vi "WPI_SimpleGyro_Loop.vi"(8 "error in":errorcluster, 11 "SimpleGyroDevRef":T1 {"Sample Rate" min=0.25 max=100.0 step=0.25}) -> (0 "error out":errorcluster)   [LabVIEW 2015, in "FRC Gyro and Accel.lvlib"]
doc: "Periodically reads the SimpleGyro and makes data available to your robot project. Place this block within PeriodicTasks.vi."
uses:
  FRC Gyro and Accel.lvlib
  WPI_SimpleGyroDevRef.ctl
  <vilib>/Rock Robotics/SystemInterfaces/spilib/spi_bus.ctl
  <vilib>/Rock Robotics/WPI/SPI/WPI_SPIDevRef.ctl
  <vilib>/Platform/TimedLoop/XDataNode/timing_clust.ctl
  <vilib>/Platform/TimedLoop/XDataNode/nitl_modes.ctl
  <vilib>/Platform/TimedLoop/XDataNode/wakeup.ctl
  <vilib>/platform/TimedLoop/XDataNode/XDataNode.xnode
  <vilib>/Platform/TimedLoop/XDataNode/XDNodeRunTimeDep.lvlib
  <vilib>/ptbypt/NI_PtbyPt.lvlib
panel:
  out "Rate":dbl
  out "Device Found":bool
  out "Offset":dbl
  out "mean 2":dbl format="%0.2f"
  out "Angle":dbl
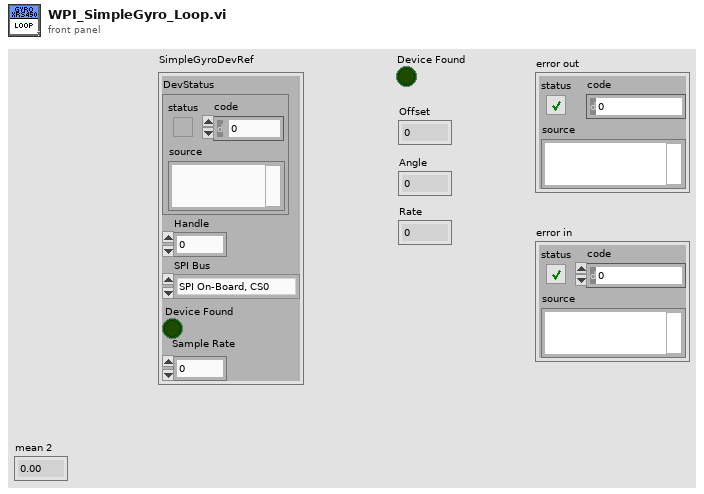
[diagram p1: front panel]
types:
  T1 = typedef "FRC Gyro and Accel.lvlib/WPI_SimpleGyroDevRef.ctl" = cluster{"DevStatus":errorcluster, "Handle":i32, "SPI Bus":T2, "Device Found":bool, "Sample Rate":dbl}
  T2 = typedef "spi_bus.ctl" = enum16{"SPI On-Board, CS0", "SPI On-Board, CS1", "SPI On-Board, CS2", "SPI On-Board, CS3", "SPI MXP", "Invalid"}
  T3 = typedef "WPI_SPIDevRef.ctl" = cluster{"DevStatus":errorcluster, "Handle":i32, "SPI Bus":T2}
  T4 = typedef "XDNodeRunTimeDep.lvlib/timing_clust.ctl" = cluster{"Expected End [f-1]":u64, "Actual End [f-1]":u64, "Finished Late? [f-1]":bool, "Expected End [i-1]":u64, "Actual End [i-1]":u64, "Finished Late? [i-1]":bool, "Expected Start [i]":u64, "Actual Start [i]":u64, "Expected Start [f]":u64, "Actual Start [f]":u64, "Source Name":string, "Structure Name":string, "Period":i64, "Deadline":i64, "Offset":i64, "Start":i64, "Priority":i32, "Timeout":i32, "Mode":T5, "Wakeup Reason":T6, "Error":errorcluster, "Source Type":string, "Secondary Source Type":string, "Global End Time":u64, "Global Start Time":u64, "Frame Duration":u64, "Iteration Duration":u64, "Assigned CPU":i32, "I/O Scan Engine Mode":u32}
  T5 = typedef "XDNodeRunTimeDep.lvlib/nitl_modes.ctl" = enum32{"No Change", "Process missed periods, maintain original phase", "Discard missed periods, maintain original phase", "Process missed periods, ignore original phase", "Discard missed periods, ignore original phase"}
  T6 = typedef "XDNodeRunTimeDep.lvlib/wakeup.ctl" = enum32{"Normal", "Aborted", "Asynchronous wakeup", "Timing source error", "Timed loop error", "Timeout"}
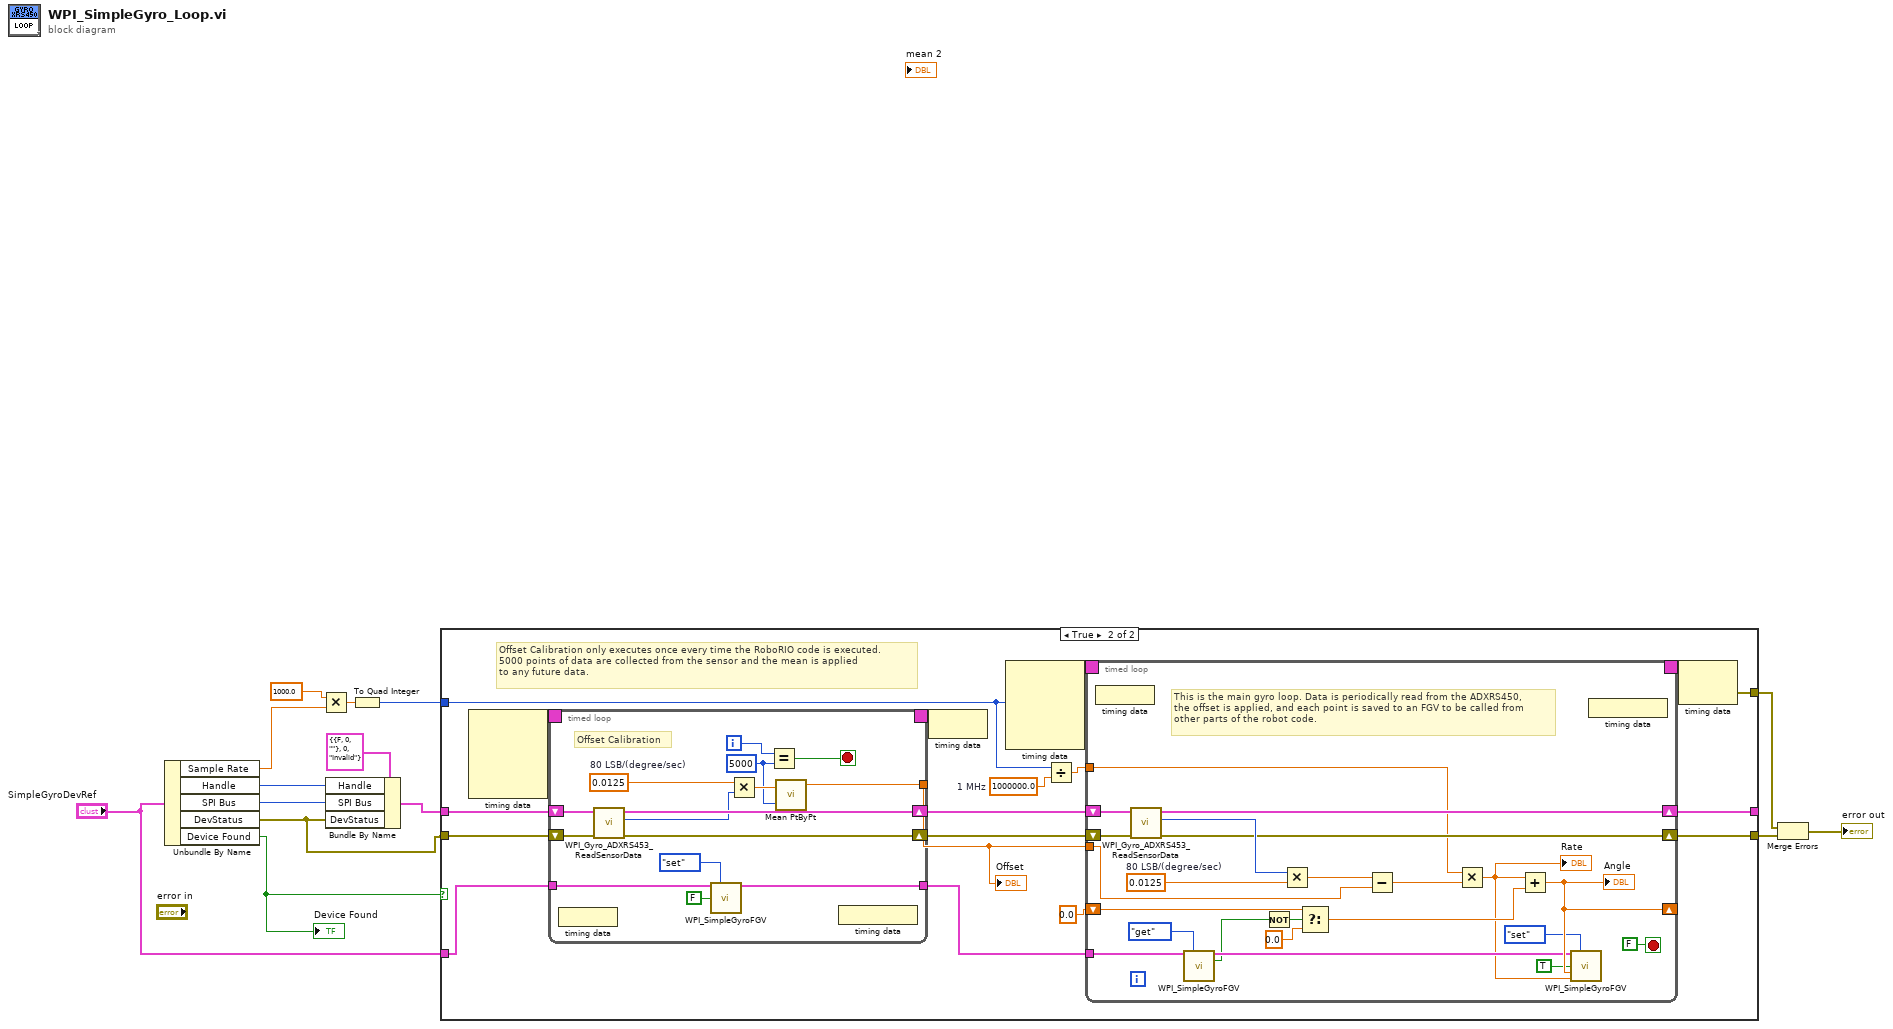
[diagram p0: block diagram]
diagram:
  n1 = Unbundle By Name("SimpleGyroDevRef") -> ("Sample Rate"=w4:dbl, "Handle"=w13:i32, "SPI Bus"=w12:T2, "DevStatus"=w1:errorcluster, "Device Found"=w11:bool)
  "Device Found" <- w11
  n2 = Multiply(x=1000.0 ("y"), y=w4) -> (x*y=w10:dbl)
  n3 = Bundle By Name(cluster=T3 {"DevStatus"={"status"=FALSE, "code"=0, "source"=""}, "Handle"=0, "SPI Bus"=enum."Invalid"} ("SPIDevRef out"), "Handle"=w13, "SPI Bus"=w12, "DevStatus"=w1) -> (w2:T3)
  n4 = To Quad Integer(1:w10) -> (0:w9:i64)
  n5 = case shown="True" w11 {
    tunnel: w2 -> [w16 w23]
    tunnel: w1 -> [w15 w22]
    tunnel: [w15 w32] -> w7
    tunnel: [w16 w31] -> _
    tunnel: w9 -> [_ w29]
    tunnel: "SimpleGyroDevRef" -> [_ w18]
    tunnel: [_ w28] -> w6
    frame False {
    }
    frame True {
      w26 = 1000000.0  # 1 MHz
      # "Offset Calibration only executes once every time the RoboRIO code is executed.\n5000 points of data are collected from the sensor and the mean is applied\nto any future data."
      n6 = node-c288() -> (w25:T4)  [unwired: 4 in]
      n7 = timed-loop {
        shift-right: [w47] -> w21
        shift-left: w23 -> [w49]
        shift-right: [w44] -> w20
        shift-left: w22 -> [w48]
        timing: w25 -> [_]
        timing-out: [_] -> w24
        tunnel: [w42] -> w19
        tunnel: w18 -> [w37]
        tunnel: [w35] -> w17
        i -> [w41]
        stop <- w39 stop-if-true
        w40 = 5000 ("y")
        w45 = 0.0125  # 80 LSB/(degree/sec)
        # "Offset Calibration"
        n8 = node-c288() -> ()  [unwired: 1 in]
        n9 = call "WPI_Gyro_ADXRS453_ReadSensorData.vi"("error in (no error)"=w48, "SPIDevRef in"=w49) -> ("error out"=w44:errorcluster, "Sensor Data (n-1)"=w46:i16, "SPIDevRef out"=w47:T3)  [unwired: 5 in, 2 out]
        n10 = call "WPI_SimpleGyroFGV.vi"("SimpleGyroDevRef"=w37, "Operation"=enum16{"set", "get"}."set", "Calibrated"=FALSE) -> ("SimpleGyroDevRef"=w35:T1)  [unwired: 8 in, 4 out]
        n11 = Multiply(x=w45, y=w46) -> (x*y=w43:dbl)
        n12 = Equal?(x=w41, y=w40) -> (x = y?=w39:bool)
        n13 = call <vilib>:"Mean PtByPt.vi"("x"=w43, "sample length"=w40) -> ("mean"=w42:dbl)  [unwired: 2 in, 1 out]
        n14 = node-c288() -> ()  [unwired: 1 out]
      }
      "Offset" <- w19
      n15 = node-c288(w24) -> ()
      n16 = node-c288(w29) -> (w34:T4)  [unwired: 3 in]
      n17 = Divide(x=w29, y=w26) -> (x/y=w30:dbl)
      n18 = timed-loop {
        shift-right: [w74] -> w31
        shift-left: w21 -> [w76]
        shift-right: [w70] -> w32
        shift-left: w20 -> [w75]
        timing: w34 -> [_]
        timing-out: [_] -> w33
        shift-right: [w63] -> _
        shift-left: 0.0 -> [w71]
        tunnel: w30 -> [w59]
        tunnel: w17 -> [w65]
        tunnel: w19 -> [w57]
        stop <- FALSE stop-if-true
        w72 = 0.0125  # 80 LSB/(degree/sec)
        # "This is the main gyro loop. Data is periodically read from the ADXRS450, \nthe offset is applied, and each point is saved to an FGV to be called from\nother parts of the robot code."
        n19 = node-c288() -> ()  [unwired: 1 in]
        n20 = call "WPI_Gyro_ADXRS453_ReadSensorData.vi"("error in (no error)"=w75, "SPIDevRef in"=w76) -> ("error out"=w70:errorcluster, "Sensor Data (n-1)"=w73:i16, "SPIDevRef out"=w74:T3)  [unwired: 5 in, 2 out]
        n21 = call "WPI_SimpleGyroFGV.vi"("SimpleGyroDevRef"=w65, "Operation"=enum16{"set", "get"}."get") -> ("SimpleGyroDevRef"=w61:T1, "Reset?"=w60:bool)  [unwired: 9 in, 3 out]
        n22 = Not(x=w60) -> (.not. x?=w66:bool)
        n23 = Multiply(x=w73, y=w72) -> (x*y=w58:dbl)
        n24 = Select(t=w71, s=w66, f=0.0 ("t")) -> (s? t:f=w68:dbl)
        n25 = Subtract(x=w58, y=w57) -> (x-y=w56:dbl)
        n26 = Multiply(x=w59, y=w56) -> (x*y=w55:dbl)
        "Rate" <- w55
        n27 = Add(x=w55, y=w68) -> (x+y=w63:dbl)
        "Angle" <- w63
        n28 = call "WPI_SimpleGyroFGV.vi"("SimpleGyroDevRef"=w61, "Operation"=enum16{"set", "get"}."set", "Calibrated"=TRUE, "Angle"=w63, "Rate"=w55) -> ()  [unwired: 6 in, 5 out]
        n29 = node-c288() -> ()  [unwired: 1 out]
      }
      n30 = node-c288(w33) -> (w28:errorcluster)
    }
  }
  n31 = Merge Errors(w6, w7) -> (→"error out":errorcluster)
